vi "Launch-lasing.vi"(8 "error in (no error)":errorcluster, 11 "Object ref in":T1) -> (0 "error out":errorcluster, 1 "Succes?":bool, 3 "Object ref out":T1)   [LabVIEW 2013, in "SLMControl.lvlib" / "SC-Main.lvclass"]
uses:
  SC-Main.lvclass
  Object-reference.ctl
  UI/Control-names.ctl
  Vision-actions.ctl
  SC-Main.lvclass/SC-Main.ctl
  Read UI.vi
  Read Lasing control.vi
  UI/Set-control-boolean.vi
  UI/SC-UI.lvclass
  SM1000/SM1000.lvclass
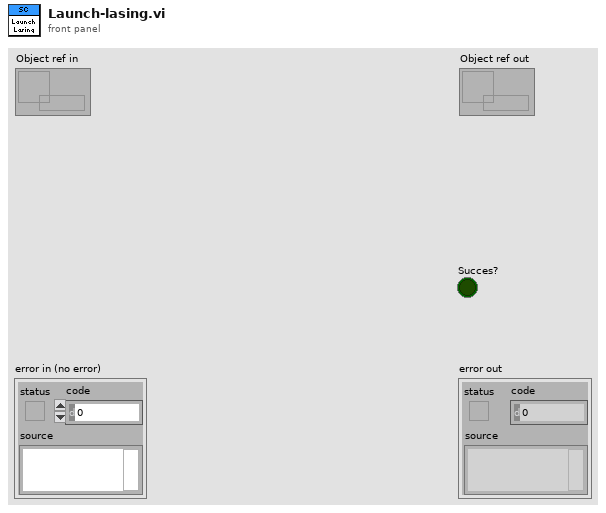
[diagram p1: front panel]
types:
  T1 = typedef "SLMControl.lvlib/SC-Main.lvclass/Object-reference.ctl" = refnum<data-value>
  T2 = typedef "SLMControl.lvlib/SC-Main.lvclass/Vision-actions.ctl" = enum16{"Activate", "Start", "Repeat", "Stop", "Exit"}
  T3 = typedef "SLMControl.lvlib/SC-UI.lvclass/Control-names.ctl" = enum16{"Com-in", "Com-out", "Help", "Status", "Load configuration", "Save configuration", "Load lasing files", "Load deposition files", "Clear", "Files", "Activate", "Execute", "Abort", "Options", "Current layer", "Current iteration", "Last elapsed time", "Deposition status", "Lasing job", "Status LEDs", "Exiting led", "Initialized led", "Files loaded led", "Activated led", "Executing led", "Deposition led", "Lasing job led", "Lasing led"}
  T4 = typedef "SLMControl.lvlib/SC-UI.lvclass/Panes-reference.ctl" = refnum<data-value>
  T5 = typedef "SLMControl.lvlib/SM1000.lvclass/Object-reference.ctl" = refnum<data-value>
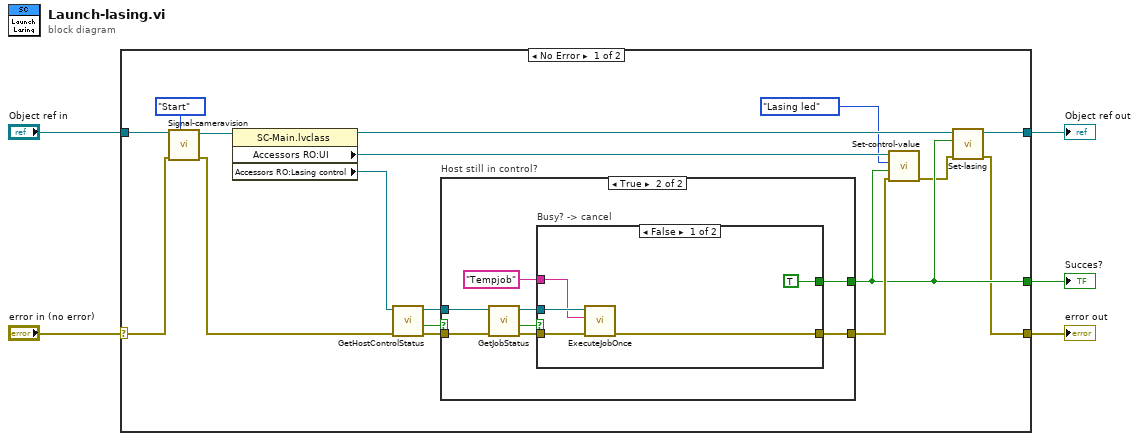
[diagram p0: block diagram]
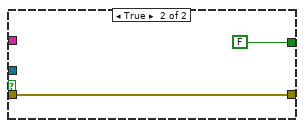
[diagram p3: hidden frame]
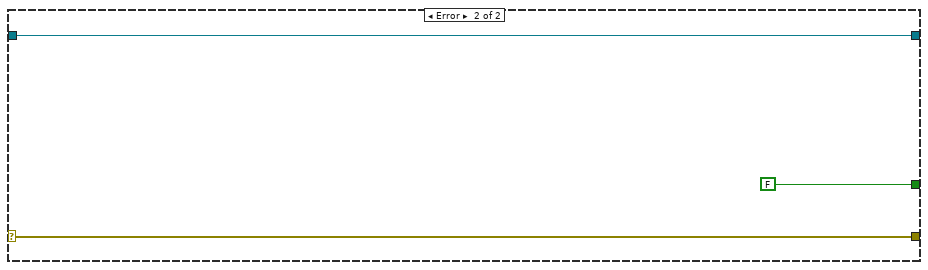
[diagram p4: hidden frame]
diagram:
  n1 = case shown="No Error" "error in (no error)" {
    selector: "error in (no error)" -> [w7 w41]
    tunnel: [w15 w41] -> w4
    tunnel: [w18 w40] -> w2
    tunnel: "Object ref in" -> [w9 w40]
    tunnel: [w17 FALSE] -> w1
    frame No Error {
      n2 = call "Signal-cameravision.vi"("Vision action"=Vision-actions."Start", "error in (no error)"=w7, "Object ref in"=w9) -> ("error out"=w6:errorcluster, "Object ref out"=w8:T1)  [unwired: 7 in]
      n3 = property class="SC-Main.lvclass"(reference=w8) -> (reference out=w22:T1, "Accessors RO:UI"=w21:T4, "Accessors RO:Lasing control"=w12:T5)  [unwired: 1 in, 1 out]
      n4 = call "GetHostControlStatus.vi"("error in (no error)"=w6, "SM1000-control in"=w12) -> ("error out"=w14:errorcluster, "Host in control?"=w11:bool, "SM1000-control out"=w13:T5)  [unwired: 7 in]
      n5 = case "Host still in control?" shown="True" w11 {
        tunnel: [w23 w28] -> w19
        tunnel: [_ w26] -> w17
        tunnel: w14 -> [w23 w25]
        tunnel: w13 -> [_ w24]
        frame False {
        }
        frame True {
          n6 = call "GetJobStatus.vi"("error in (no error)"=w25, "SM1000-control in"=w24) -> ("error out"=w31:errorcluster, "Busy?"=w29:bool, "SM1000-control out"=w30:T5)  [unwired: 7 in]
          n7 = case "Busy? -> cancel" shown="False" w29 {
            tunnel: w31 -> [w36 w38]
            tunnel: w30 -> [w35 _]
            tunnel: [w32 w38] -> w28
            tunnel: [TRUE FALSE] -> w26
            tunnel: "Tempjob" -> [w34 _]
            frame False {
              n8 = call "ExecuteJobOnce.vi"("error in (no error)"=w36, "Job name wo extension"=w34, "SM1000-control in"=w35) -> ("error out"=w32:errorcluster)  [unwired: 7 in, 1 out]
            }
            frame True {
            }
          }
        }
      }
      n9 = call-poly "Set-control-value.vi"("error in (no error)"=w19, "Value"=w17, "Control name"=Control-names."Lasing led", "Panes in"=w21) -> ("error out"=w16:errorcluster)  [unwired: 6 in, 1 out]
      n10 = call "Set-lasing.vi"("error in (no error)"=w16, "Lasing?"=w17, "Object ref in"=w22) -> ("error out"=w15:errorcluster, "Object ref out"=w18:T1)  [unwired: 7 in]
    }
    frame Error {
    }
  }
  "error out" <- w4
  "Object ref out" <- w2
  "Succes?" <- w1
